vi "get_new_control_position.vi"(9 "control bounds":cluster{"Width":u32, "Height":u32}, 10 "control postion":cluster{"Left":i32, "Top":i32}, 11 "mouse position":cluster{"Horizontal":i32, "Vertical":i32}) -> (1 "in range":bool, 2 "control postion new":cluster{"Left":i32, "Top":i32})   [LabVIEW 2021, in "FirstXNode .xnode"]
uses:
  FirstXNode .xnode
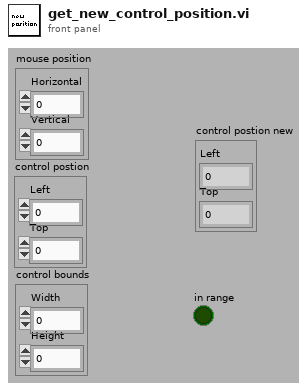
[diagram p1: front panel]
types:
  T1 = enum16{"to left", "to top", "to right", "to bottom"}
  T2 = cluster{dbl, enum16{"to left", "to top", "to right", "to bottom"}}
  T3 = cluster{dbl, enum16{"to left", "to top", "to right", "to bottom"}}[]
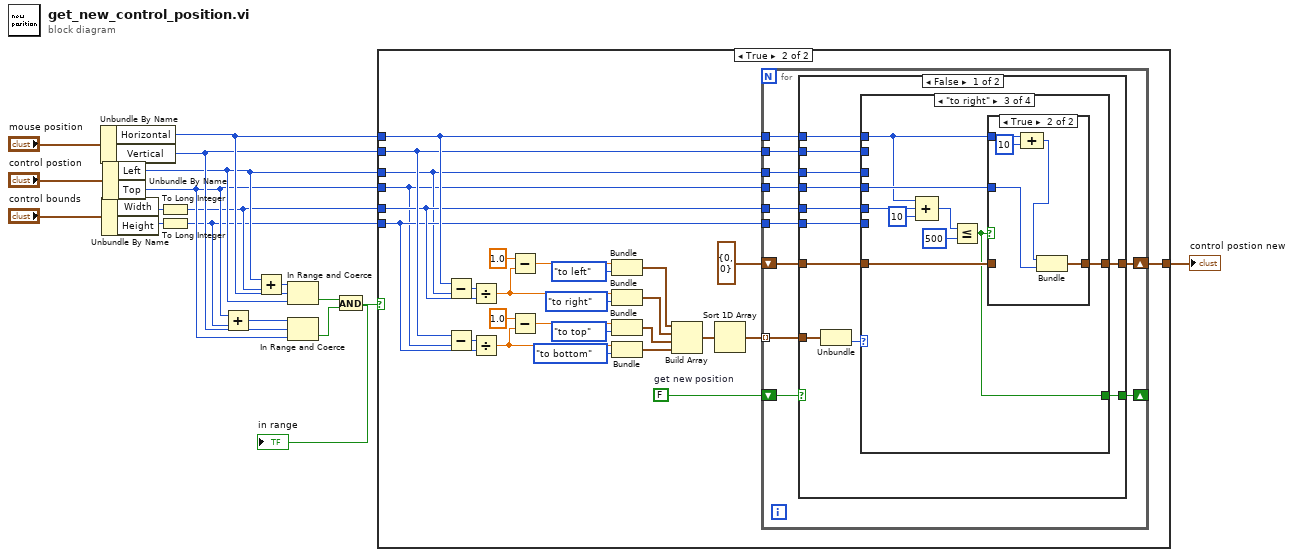
[diagram p0: block diagram]
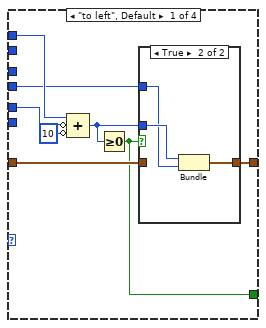
[diagram p3: hidden frame]
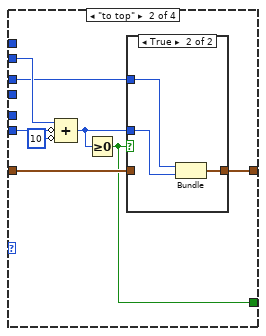
[diagram p5: hidden frame]
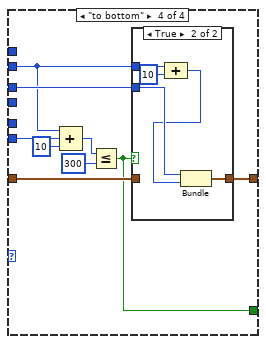
[diagram p8: hidden frame]
diagram:
  n1 = Unbundle By Name("mouse position") -> ("Horizontal"=w9:i32, "Vertical"=w8:i32)
  n2 = Unbundle By Name("control bounds") -> ("Width"=w5:u32, "Height"=w4:u32)
  n3 = Unbundle By Name("control postion") -> ("Left"=w7:i32, "Top"=w6:i32)
  n4 = To Long Integer(number=w5) -> (32bit integer=w3:i32)
  n5 = To Long Integer(number=w4) -> (32bit integer=w2:i32)
  n6 = Add(x=w6, y=w2) -> (x+y=w15:i32)
  n7 = Add(x=w7, y=w3) -> (x+y=w14:i32)
  n8 = In Range and Coerce(upper limit=w14, x=w9, lower limit=w7) -> (In Range?=w16:bool)  [unwired: 1 out]
  n9 = In Range and Coerce(upper limit=w15, x=w8, lower limit=w6) -> (In Range?=w17:bool)  [unwired: 1 out]
  n10 = And(x=w16, y=w17) -> (x .and. y?=w10:bool)
  "in range" <- w10
  n11 = case shown="True" w10 {
    tunnel: w9 -> [_ w25]
    tunnel: w8 -> [_ w24]
    tunnel: w7 -> [_ w20]
    tunnel: w6 -> [_ w19]
    tunnel: w3 -> [_ w23]
    tunnel: w2 -> [_ w22]
    tunnel: [_ w18] -> w1
    frame False {
    }
    frame True {
      w26 = FALSE  # get new position
      n12 = Subtract(x=w25, y=w20) -> (x-y=w44:i32)
      n13 = Subtract(x=w24, y=w19) -> (x-y=w43:i32)
      n14 = Divide(x=w44, y=w23) -> (x/y=w37:dbl)
      n15 = Divide(x=w43, y=w22) -> (x/y=w33:dbl)
      n16 = Subtract(x=1.0, y=w37) -> (x-y=w40:dbl)
      n17 = Subtract(x=1.0, y=w33) -> (x-y=w35:dbl)
      n18 = Bundle(w40, T1."to left") -> (w32:T2)  [unwired: 1 in]
      n19 = Bundle(w37, T1."to right") -> (w31:T2)  [unwired: 1 in]
      n20 = Bundle(w35, T1."to top") -> (w30:T2)  [unwired: 1 in]
      n21 = Bundle(w33, T1."to bottom") -> (w29:T2)  [unwired: 1 in]
      n22 = Build Array(w32, w31, w30, w29) -> (w28:T3)
      n23 = Sort 1D Array(array=w28) -> (sorted array=w27:T3)
      n24 = for {
        tunnel: w27 -> [w54] mode=indexing
        shift-right: [w45] -> _
        shift-left: w26 -> [w55]
        tunnel: w25 -> [w53]
        tunnel: w24 -> [w52]
        tunnel: w23 -> [w51]
        tunnel: w22 -> [w50]
        shift-right: [w48] -> w18
        shift-left: cluster{"Left":i32, "Top":i32} {"Left"=0, "Top"=0} ("control postion") -> [w47]
        tunnel: w20 -> [w49]
        tunnel: w19 -> [w46]
        n25 = case shown="False" w55 {
          selector: w55 -> [_ w121]
          tunnel: w54 -> [w66 _]
          tunnel: w53 -> [w63 _]
          tunnel: w52 -> [w64 _]
          tunnel: w51 -> [w62 _]
          tunnel: w50 -> [w61 _]
          tunnel: w49 -> [w60 _]
          tunnel: [w59 w122] -> w48
          tunnel: w47 -> [w58 w122]
          tunnel: w46 -> [w57 _]
          tunnel: [w56 w121] -> w45
          frame False {
            n26 = Unbundle(w66) -> (w65:T1)  [unwired: 1 out]
            n27 = case shown="\"to right\"" w65 {
              tunnel: w64 -> [_ w86 _ w106]
              tunnel: w63 -> [w72 _ w91 _]
              tunnel: w62 -> [w68 _ w98 _]
              tunnel: w61 -> [_ w85 _ w110]
              tunnel: w60 -> [_ w83 _ w111]
              tunnel: [w69 w81 w94 w112] -> w59
              tunnel: w58 -> [w70 w80 w95 w113]
              tunnel: w57 -> [w71 _ w93 _]
              tunnel: [w67 w79 w92 w107] -> w56
              frame "to left", Default {
                n28 = Compound Arithmetic op=ADD(w72, invert w68, invert 10 ("value")) -> (w73:i32)
                n29 = Greater Or Equal To 0?(x=w73) -> (x >= 0?=w67:bool)
                n30 = case shown="True" w67 {
                  tunnel: w73 -> [_ w77]
                  tunnel: [w75 w78] -> w69
                  tunnel: w70 -> [w75 _]
                  tunnel: w71 -> [_ w76]
                  frame False {
                  }
                  frame True {
                    n31 = Bundle(w77, "Top"=w76) -> (w78:cluster{i32, "Top":i32})  [unwired: 1 in]
                  }
                }
              }
              frame "to top" {
                n32 = Compound Arithmetic op=ADD(w86, invert w85, invert 10 ("value")) -> (w82:i32)
                n33 = Greater Or Equal To 0?(x=w82) -> (x >= 0?=w79:bool)
                n34 = case shown="True" w79 {
                  tunnel: w83 -> [_ w90]
                  tunnel: w82 -> [_ w89]
                  tunnel: [w87 w88] -> w81
                  tunnel: w80 -> [w87 _]
                  frame False {
                  }
                  frame True {
                    n35 = Bundle("Left"=w90, w89) -> (w88:cluster{"Left":i32, i32})  [unwired: 1 in]
                  }
                }
              }
              frame "to right" {
                n36 = Compound Arithmetic op=ADD(w91, w98, 10 ("value")) -> (w97:i32)
                n37 = Less Or Equal?(x=w97, y=500) -> (x <= y?=w92:bool)
                n38 = case shown="True" w92 {
                  tunnel: w93 -> [_ w104]
                  tunnel: [w100 w105] -> w94
                  tunnel: w95 -> [w100 _]
                  tunnel: w91 -> [_ w103]
                  frame False {
                  }
                  frame True {
                    n39 = Compound Arithmetic op=ADD(w103, 10 ("value")) -> (w101:i32)
                    n40 = Bundle(w101, "Top"=w104) -> (w105:cluster{i32, "Top":i32})  [unwired: 1 in]
                  }
                }
              }
              frame "to bottom" {
                n41 = Compound Arithmetic op=ADD(w106, w110, 10 ("value")) -> (w108:i32)
                n42 = Less Or Equal?(x=w108, y=300) -> (x <= y?=w107:bool)
                n43 = case shown="True" w107 {
                  tunnel: w111 -> [_ w120]
                  tunnel: [w115 w119] -> w112
                  tunnel: w113 -> [w115 _]
                  tunnel: w106 -> [_ w117]
                  frame False {
                  }
                  frame True {
                    n44 = Compound Arithmetic op=ADD(w117, 10 ("value")) -> (w116:i32)
                    n45 = Bundle("Left"=w120, w116) -> (w119:cluster{"Left":i32, i32})  [unwired: 1 in]
                  }
                }
              }
            }
          }
          frame True {
          }
        }
      }
    }
  }
  "control postion new" <- w1
